vi "Configure Alarm Output.vi"(0 "VISA resource name":refnum<visa-resource-name>, 1 "Unit Address (1)":i16=1, 2 "Latching (0: Alarm Self-Clears)":u16(ring) items=["Alarm Self-Clears", "Alarm Latches"], 3 "Silencing (F: No)":bool, 5 "Alarm Output (1)":i16=1, 7 "Alarm Hysteresis (3.0)":dbl=3.0 format="%.2f", 9 "Alarm Sides (0: Both)":u16(ring) items=["Both", "Low", "High"], 11 "error in (no error)":errorcluster {"code" format="%.0x"}, 12 "Alarm Logic (0: Open On Alarm)":u16(ring) items=["Open On Alarm", "Close On Alarm"], 13 "Alarm Messages (0: Yes on Main Page)":u16(ring) items=["Yes on Main Page", "No"]) -> (4 "VISA resource name out":refnum<visa-resource-name>, 15 "error out":errorcluster {"code" format="%.0x"})   [LabVIEW 2010]
doc: "This VI configures alarm output."
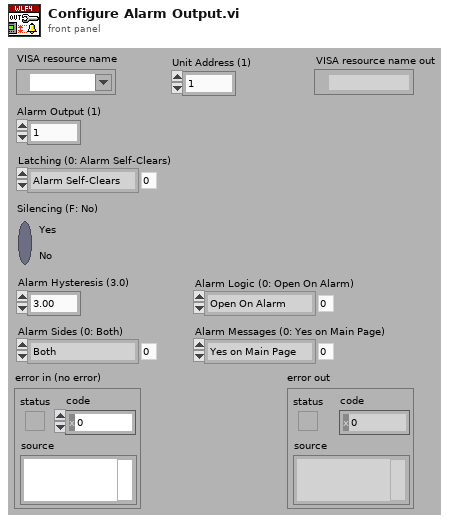
[diagram p1: front panel]
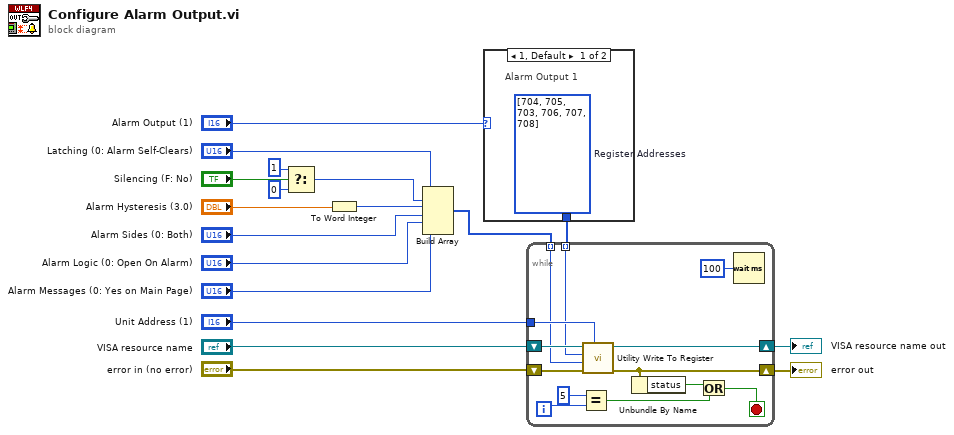
[diagram p0: block diagram]
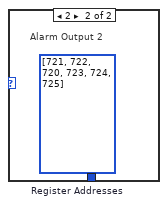
[diagram p2: hidden frame]
diagram:
  n1 = Select(t=1, s="Silencing (F: No)", f=0) -> (s? t:f=w8:i32)
  n2 = To Word Integer(number="Alarm Hysteresis (3.0)") -> (16bit integer=w1:i16)
  n3 = Build Array("Latching (0: Alarm Self-Clears)", w8, w1, "Alarm Sides (0: Both)", "Alarm Logic (0: Open On Alarm)", "Alarm Messages (0: Yes on Main Page)") -> (w13:i32[])
  n4 = case shown="1, Default" "Alarm Output (1)" {
    tunnel: [w19 w20] -> w15
    frame 1, Default {
      w19 = i32[] [704, 705, 703, 706, 707, 708]  # Register Addresses
      # "Alarm Output 1"
    }
    frame 2 {
      w20 = i32[] [721, 722, 720, 723, 724, 725]  # Register Addresses
      # "Alarm Output 2"
    }
  }
  n5 = while {
    tunnel: "Unit Address (1)" -> [w33]
    shift-right: [w30] -> w18
    shift-left: "VISA resource name" -> [w32]
    shift-right: [w26] -> w17
    shift-left: "error in (no error)" -> [w31]
    tunnel: w15 -> [w28] mode=indexing
    tunnel: w13 -> [w27] mode=indexing
    i -> [w23]
    stop <- w25 stop-if-true
    n6 = Equal?(x=5, y=w23) -> (x = y?=w21:bool)
    n7 = call "Utility Write To Register.vi"("Unit Address (1)"=w33, "error in (no error)"=w31, "Data (0)"=w27, "Register Address (0)"=w28, "VISA resource name"=w32) -> ("error out"=w26:errorcluster, "VISA resource name out"=w30:refnum<visa-resource-name>)  [unwired: 5 in]
    n8 = Unbundle By Name(w26) -> ("status"=w24:bool)
    n9 = Or(x=w24, y=w21) -> (x .or. y?=w25:bool)
    n10 = Wait (ms)(milliseconds to wait=u32 100) -> ()  [unwired: 1 out]
  }
  "error out" <- w17
  "VISA resource name out" <- w18
